vi "Destroy.vi"(8 "Error In":errorcluster) -> (0 "Error Out":errorcluster, 2 "No. Of Remaining Elements":i32, 3 "Remaining Elements":T1[](array[typedef]))   [LabVIEW 2023, in "Error Manager.lvlib" / "New Error Window.lvlib" / "MHL Queue.lvlib"]
doc: "Destroys (or releases) the queue. (Force Destroy is set to TRUE.)"
uses:
  MHL Queue.lvlib
  Message (cluster).ctl
  Command (enum).ctl
  Queue Reference (library variable).vi
panel:
  # "Input\nInputs to the VI"
  # "Development\nControls or indicators that are useful for development or testing, but which are not outputs of the VI."
  # "Output\nOutputs of the VI"
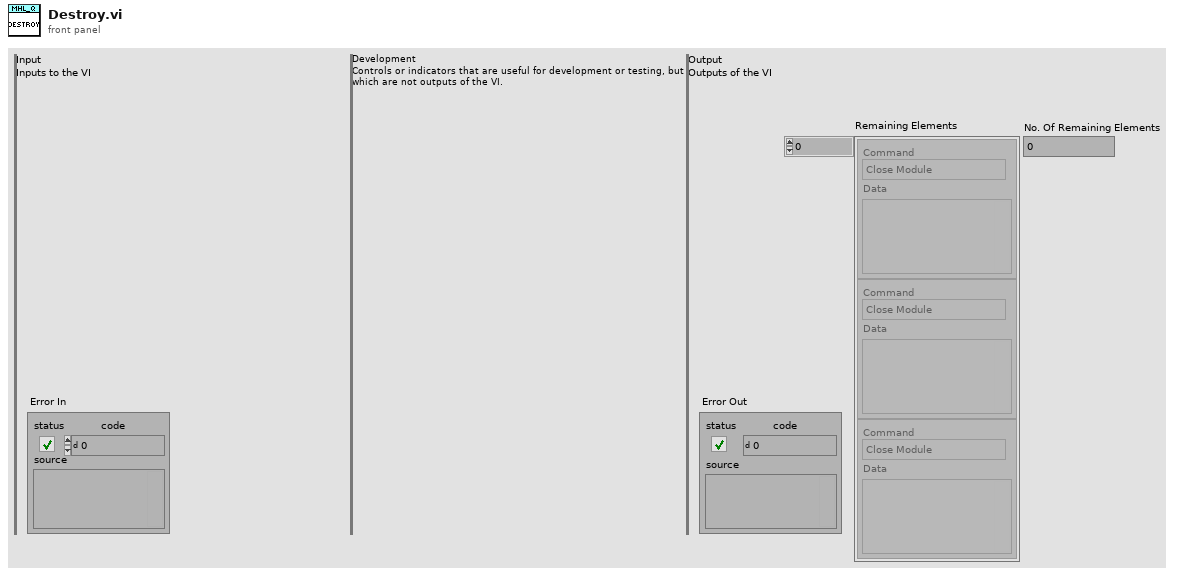
[diagram p1: front panel]
types:
  T1 = typedef "Error Manager.lvlib/New Error Window.lvlib/MHL Queue.lvlib/Message (cluster).ctl" = cluster{"Command":T2, "Data":variant}
  T2 = typedef "Error Manager.lvlib/New Error Window.lvlib/MHL Queue.lvlib/Command (enum).ctl" = enum16{"Init Module", "Close Module", "Handle Local Error", "OK Button Pressed"}
  T3 = typedef "Error Manager.lvlib/New Error Dialogue GUI.lvlib/MHL Queue.lvlib/Message (cluster).ctl" = cluster{"Command":T4, "Data":variant}
  T4 = typedef "Error Manager.lvlib/New Error Dialogue GUI.lvlib/MHL Queue.lvlib/Command (enum).ctl" = enum16{"Init Module", "Close Module", "Handle Local Error", "OK Button Pressed"}
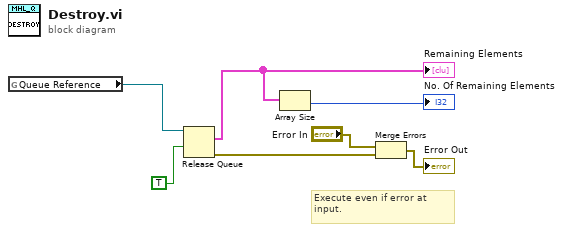
[diagram p0: block diagram]
diagram:
  # "Execute even if error at input."
  n1 = global read "Queue Reference (library variable).vi" "Queue Reference"() -> (w1:refnum<queue>)
  n2 = Release Queue(queue=w1, force destroy? (F)=TRUE) -> (remaining elements=w3:T3[], error out=w7:errorcluster)  [unwired: 1 in, 1 out]
  "Remaining Elements" <- w3
  n3 = Array Size(array=w3) -> (size(s)=→"No. Of Remaining Elements":i32)
  n4 = Merge Errors("Error In", w7) -> (→"Error Out":errorcluster)
